vi "Workspace.UI.DisableState.Set.vi"(7 "Enable?":bool=TRUE, 8 "error in (no error)":errorcluster, 11 "State Variables in":T1) -> (0 "error out":errorcluster, 3 "State Variables out":T1)   [LabVIEW 2019, in "Diagnostics Workspace Shared.lvlib"]
uses:
  Diagnostics Workspace Shared.lvlib
  Types/Workspace.State.ctl
  Addon/Addon Shared/Types/UI.Refs.ctl
  Addon/Addon Shared/Types/Command.New.ctl
  SubModules/CAN-Streaming-Support/Addon/Addon Shared/Types/Type Filter.ctl
  <vilib>/NI VeriStand/Display Template Support/DisplayTemplateSupport.llb/enum_Display Template Handler Minimal To Workspace.ctl
  Types/Workspace.SavedState.ctl
  NationalInstruments.VeriStand.SystemStorage
  <vilib>/NI VeriStand/Execution/Workspace/WorkspaceAPI.ctl
  NationalInstruments.VeriStand.ClientAPI
  <vilib>/NI VeriStand/Display Template Support/DisplayTemplateSupport.llb/enum_Display Template Handler Minimal To Widget Msg.ctl
  <vilib>/NI VeriStand/Execution/Workspace/SystemStateRegEventRef.ctl
  <vilib>/NI VeriStand/Execution/Workspace/Target State Info.ctl
  <vilib>/NI VeriStand/Execution/Workspace/Target State.ctl
  <vilib>/NI VeriStand/Execution/Workspace/SystemStateEventRef.ctl
  Addon/Addon Shared/Types/Protocol.ctl
  SubModules/CAN-Streaming-Support/UIs/Workspace Shared/Types/Host Stream Queue Refs.ctl
  SubModules/CAN-Streaming-Support/UIs/Workspace Shared/Types/Host Stream Queue Type.ctl
  SubModules/CAN-Streaming-Support/UIs/Workspace Shared/Types/Host Stream Queue Command.ctl
  <vilib>/xnet/xnet.llb/XNET Frame CAN.ctl
  <vilib>/xnet/xnet.llb/XNET Frame Type CAN.ctl
  <vilib>/NI VeriStand/Execution/Workspace/NI_VS Workspace ExecutionAPI.lvlib
  Addon/Addon Shared/Diagnostics Addon Shared.lvlib
  SubModules/CAN-Streaming-Support/UIs/Workspace Shared/CAN Stream Support Workspace Shared.lvlib
  SubModules/CAN-Streaming-Support/Addon/Addon Shared/CAN Stream Support Shared.lvlib
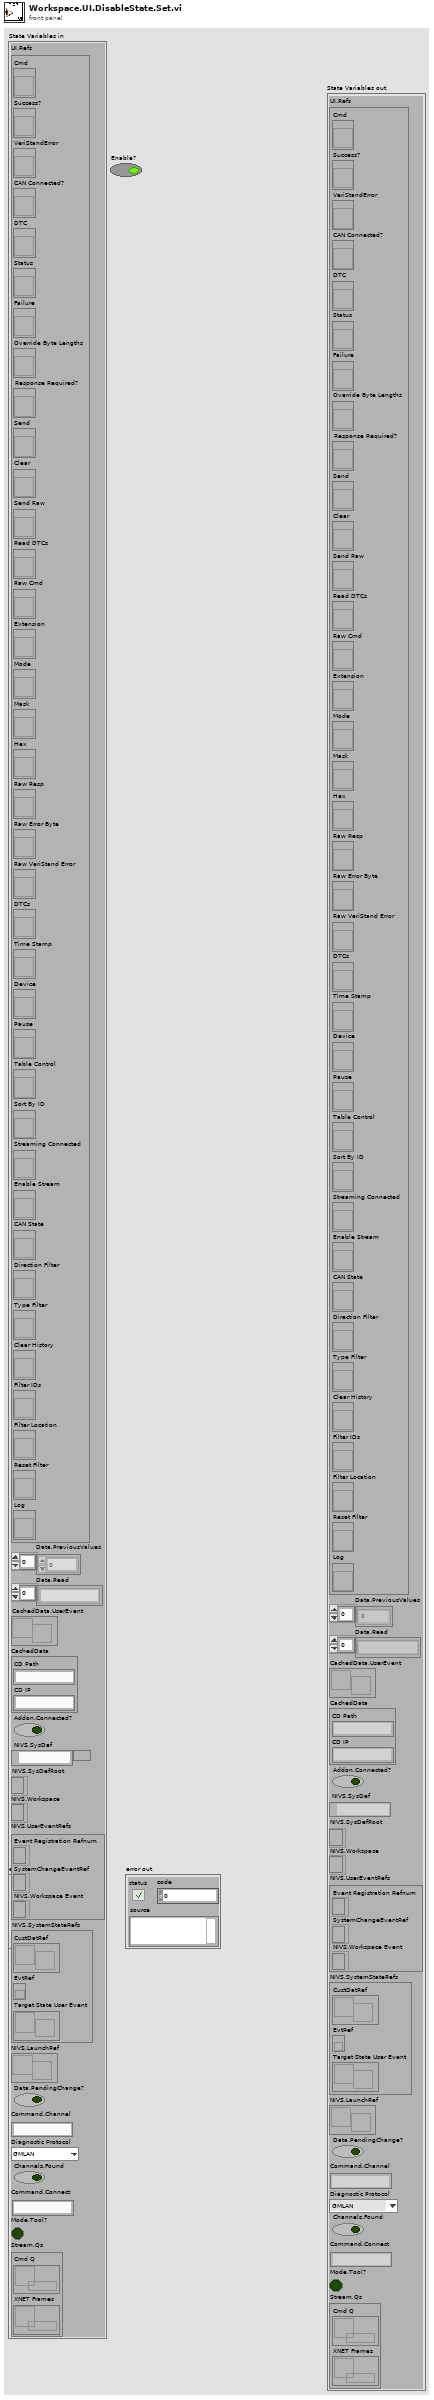
[diagram p1: front panel]
types:
  T1 = typedef "Diagnostics Workspace Shared.lvlib/Workspace.State.ctl" = cluster{"UI.Refs":T2, "Data.PreviousValues":dbl[], "Data.Read":string[], "CachedData.UserEvent":refnum<user-event>, "CachedData":T3, "Addon.Connected?":bool, "NIVS.SysDef":path, "NIVS.SysDefRoot":refnum<k24>, "NIVS.Workspace":T4, "NIVS.UserEventRefs":cluster{"Event Registration Refnum":refnum<event-registration>, "SystemChangeEventRef":T5, "NIVS.Workspace Event":refnum<event-registration>}, "NIVS.SystemStateRefs":T6, "NIVS.LaunchRef":refnum<user-event>, "Data.PendingChange?":bool, "Command.Channel":string, "Diagnostic Protocol":T7, "Channels.Found":bool, "Command.Connect":string, "Mode.Tool?":bool, "Stream.Qs":T8}
  T2 = typedef "Diagnostics Addon Shared.lvlib/UI.Refs.ctl" = cluster{"Cmd":refnum<vi>, "Success?":refnum<vi>, "VeriStandError":refnum<vi>, "CAN Connected?":refnum<vi>, "DTC":refnum<vi>, "Status":refnum<vi>, "Failure":refnum<vi>, "Override Byte Lengths":refnum<vi>, "Response Required?":refnum<vi>, "Send":refnum<vi>, "Clear":refnum<vi>, "Send Raw":refnum<vi>, "Read DTCs":refnum<vi>, "Raw Cmd":refnum<vi>, "Extension":refnum<vi>, "Mode":refnum<vi>, "Mask":refnum<vi>, "Hex":refnum<vi>, "Raw Resp":refnum<vi>, "Raw Error Byte":refnum<vi>, "Raw VeriStand Error":refnum<vi>, "DTCs":refnum<vi>, "Time Stamp":refnum<vi>, "Device":refnum<vi>, "Pause":refnum<vi>, "Table Control":refnum<vi>, "Sort By ID":refnum<vi>, "Streaming Connected":refnum<vi>, "Enable Stream":refnum<vi>, "CAN State":refnum<vi>, "Direction Filter":refnum<vi>, "Type Filter":refnum<vi>, "Clear History":refnum<vi>, "Filter IDs":refnum<vi>, "Filter Location":refnum<vi>, "Reset Filter":refnum<vi>, "Log":refnum<vi>}
  T3 = typedef "Diagnostics Workspace Shared.lvlib/Workspace.SavedState.ctl" = cluster{"CD Path":string, "CD IP":string}
  T4 = typedef "NI_VS Workspace ExecutionAPI.lvlib/WorkspaceAPI.ctl" = refnum<k24>
  T5 = typedef "NI_VS Workspace ExecutionAPI.lvlib/SystemStateRegEventRef.ctl" = refnum<event-registration>
  T6 = typedef "NI_VS Workspace ExecutionAPI.lvlib/SystemStateEventRef.ctl" = cluster{"CustDatRef":refnum<user-event>, "EvtRef":refnum<k27>, "Target State User Event":refnum<user-event>}
  T7 = typedef "Diagnostics Addon Shared.lvlib/Protocol.ctl" = enum16{"GMLAN", "KWP-2000", "UDS", "User-Defined"}
  T8 = typedef "CAN Stream Support Workspace Shared.lvlib/Host Stream Queue Refs.ctl" = cluster{"Cmd Q":refnum<queue>, "XNET Frames":refnum<queue>}
  T9 = enum8{"Enabled", "Disabled", "Disabled and Grayed Out"}
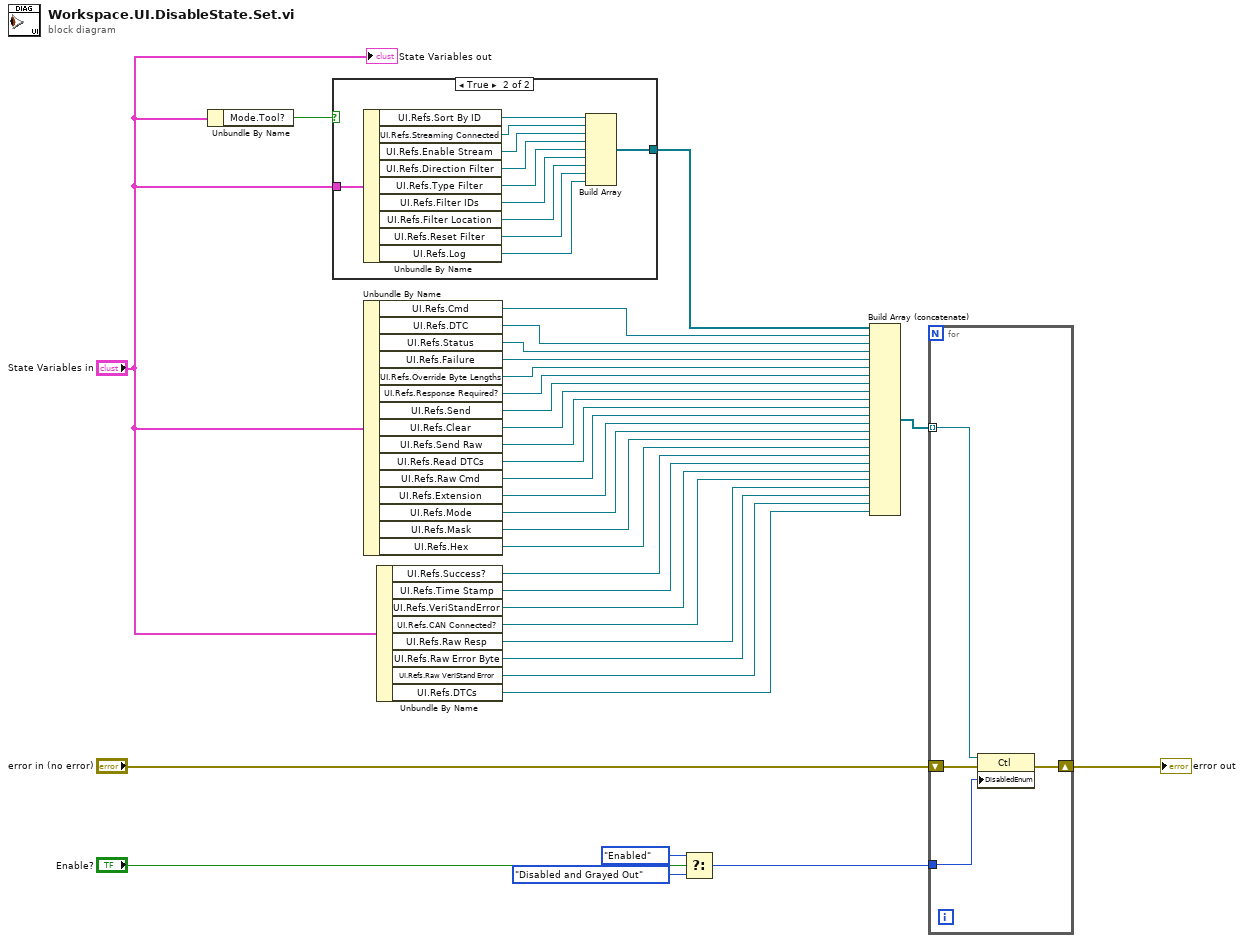
[diagram p0: block diagram]
diagram:
  n1 = Unbundle By Name("State Variables in") -> ("Mode.Tool?"=w2:bool)
  n2 = case shown="True" w2 {
    tunnel: "State Variables in" -> [_ w35]
    tunnel: [_ w34] -> w1
    frame False {
    }
    frame True {
      n3 = Unbundle By Name(w35) -> ("UI.Refs.Sort By ID"=w44:refnum<vi>, "UI.Refs.Streaming Connected"=w43:refnum<vi>, "UI.Refs.Enable Stream"=w42:refnum<vi>, "UI.Refs.Direction Filter"=w41:refnum<vi>, "UI.Refs.Type Filter"=w40:refnum<vi>, "UI.Refs.Filter IDs"=w39:refnum<vi>, "UI.Refs.Filter Location"=w38:refnum<vi>, "UI.Refs.Reset Filter"=w37:refnum<vi>, "UI.Refs.Log"=w36:refnum<vi>)
      n4 = Build Array(w44, w43, w42, w41, w40, w39, w38, w37, w36) -> (w34:refnum<vi>[])
    }
  }
  n5 = Unbundle By Name("State Variables in") -> ("UI.Refs.Cmd"=w4:refnum<vi>, "UI.Refs.DTC"=w18:refnum<vi>, "UI.Refs.Status"=w19:refnum<vi>, "UI.Refs.Failure"=w20:refnum<vi>, "UI.Refs.Override Byte Lengths"=w21:refnum<vi>, "UI.Refs.Response Required?"=w22:refnum<vi>, "UI.Refs.Send"=w23:refnum<vi>, "UI.Refs.Clear"=w24:refnum<vi>, "UI.Refs.Send Raw"=w25:refnum<vi>, "UI.Refs.Read DTCs"=w26:refnum<vi>, "UI.Refs.Raw Cmd"=w27:refnum<vi>, "UI.Refs.Extension"=w28:refnum<vi>, "UI.Refs.Mode"=w29:refnum<vi>, "UI.Refs.Mask"=w30:refnum<vi>, "UI.Refs.Hex"=w13:refnum<vi>)
  n6 = Unbundle By Name("State Variables in") -> ("UI.Refs.Success?"=w12:refnum<vi>, "UI.Refs.Time Stamp"=w11:refnum<vi>, "UI.Refs.VeriStandError"=w10:refnum<vi>, "UI.Refs.CAN Connected?"=w9:refnum<vi>, "UI.Refs.Raw Resp"=w8:refnum<vi>, "UI.Refs.Raw Error Byte"=w7:refnum<vi>, "UI.Refs.Raw VeriStand Error"=w6:refnum<vi>, "UI.Refs.DTCs"=w5:refnum<vi>)
  n7 = Select(t=T9."Enabled" ("Disabled"), s="Enable?", f=T9."Disabled and Grayed Out" ("Disabled")) -> (s? t:f=w14:T9)
  n8 = Build Array (concatenate)(w1, w4, w18, w19, w20, w21, w22, w23, w24, w25, w26, w27, w28, w29, w30, w13, w12, w11, w10, w9, w8, w7, w6, w5) -> (w31:refnum<vi>[])
  n9 = for {
    tunnel: w31 -> [w47] mode=indexing
    shift-right: [w46] -> w33
    shift-left: "error in (no error)" -> [w48]
    tunnel: w14 -> [w45]
    n10 = property class="Ctl"(reference=w47, error in=w48, "DisabledEnum"=w45) -> (error out=w46:errorcluster)  [unwired: 1 out]
  }
  "error out" <- w33
  "State Variables out" <- "State Variables in"
